vi "Pfeiffer-RVC300.reset.vi"(0 "i ref in":refnum<vi>, 3 "ms timeout (10000)":i32=10000, 5 "error in (no error)":errorcluster) -> (14 "i ref out":refnum<vi>, 19 "error out":errorcluster)   [LabVIEW 2014, in "Pfeiffer-RVC300.lvlib"]
doc: "Resets the RVC300 by closing the valve.\n\nLicense Agreement for this software:\n\nCopyright (C)\nMax-Planck-Institut für Kernphysik\nSaupfercheckweg 1\n69117 Heidelberg\nGermany\n\nContact: christopher.borgmann@mpi-hd.mpg.de\n\nThis program is free software: you can redistribute it and/or modify \nit under the terms of the GNU General Public License as published by\nthe Free Software Foundation, either version 3 of the License, or\n(at your option) any later version.\n\nThis program is distributed in the hope that it will be useful,\nbut WITHOUT ANY WARRANTY; without even the implied warranty of\nMERCHANTABILITY or FITNESS FOR A PARTICULAR PURPOSE. See the\nGNU General Public License for more details.\n\nYou should have received a copy of the GNU General Public License\nalong with this program. If not, see <http://www.gnu.org/licenses/>.\n\nMax-Planck-Institut für Kernphysik\nSaupfercheckweg 1, 69117 Heidelberg, Germany\nFor all questions and ideas contact: christopher.borgmann@mpi-hd.mpg.de\nLast update: 08.07.2010"
uses:
  Pfeiffer-RVC300.lvlib
  CSCore/CSApplicationBaseClasses/DeviceBase/DeviceBase.lvlib
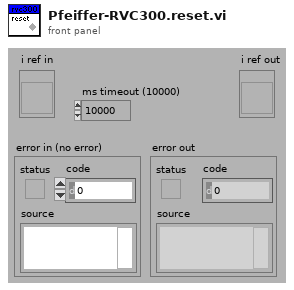
[diagram p1: front panel]
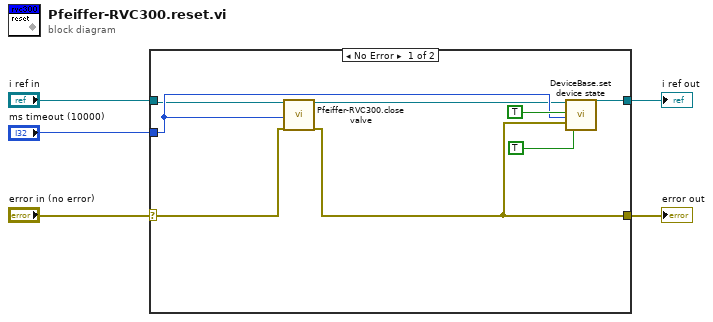
[diagram p0: block diagram]
diagram:
  n1 = case shown="No Error" "error in (no error)" {
    selector: "error in (no error)" -> [w8 w14]
    tunnel: "i ref in" -> [w7 w15]
    tunnel: [w13 w15] -> w4
    tunnel: "ms timeout (10000)" -> [w10 _]
    tunnel: [w9 w14] -> w1
    frame No Error {
      n2 = call "Pfeiffer-RVC300.close valve.vi"("i ref in"=w7, "ms timeout (10000)"=w10, "error in (no error)"=w8) -> ("i ref out"=w6:refnum<vi>, "error out"=w9:errorcluster)  [unwired: 14 in, 1 out]
      n3 = call "DeviceBase.set device state.vi"("i ref in"=w6, "implicit"=TRUE, "ms timeout (10000)"=w10, "device error"=w9, "mayResetError (FALSE)"=TRUE) -> ("i ref out"=w13:refnum<vi>)  [unwired: 12 in, 2 out]
    }
    frame Error {
    }
  }
  "error out" <- w1
  "i ref out" <- w4
